vi "Autonomous Execution.vi"(8 "error in":errorcluster, 9 "Autonomous Queue":refnum<queue>, 11 "Queue Key":refnum<queue>) -> ()   [LabVIEW 2017]
uses:
  Robot Subsystems.ctl
  Drive/Drive Notifier.ctl
  Drive/Drive Control Type.ctl
  Intake/Intake Notifier.ctl
  Intake/Intake Control Type.ctl
  Intake Rotation/Intake Rotation Notifier.ctl
  Intake Rotation/Intake Rotation Control Type.ctl
  Intake Rotation/Arm Enum States.ctl
  Lift/Lift Notifier.ctl
  Lift/Lift Control Type.ctl
  Lift/Lift Enum States.ctl
  RPED/RPED Notifier.ctl
  RPED/RPED Control Type.ctl
  Queue Key Data.ctl
panel:
  in  "ignore previous (F)":bool
  in  "timeout in ms (-1)":i32=15
  out "notifiers out":refnum<notifier>[](array[refnum])
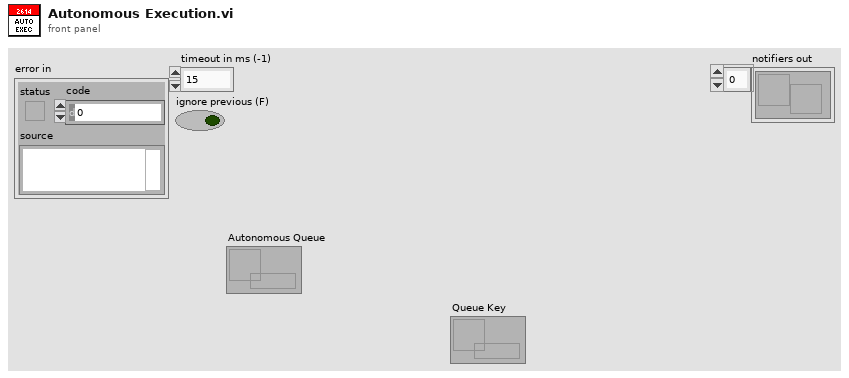
[diagram p1: front panel]
types:
  T1 = typedef "Queue Key Data.ctl" = cluster{"Operation Notifier":refnum<notifier>, "Subsystem":string, "Concurrent":bool}
  T2 = typedef "Robot Subsystems.ctl" = cluster{"Drive Notifier":T3, "Intake Notifier":T5, "Intake Rotation Notifier":T7, "Lift Notifier":T10, "RPED Notifier":T13}
  T3 = typedef "Drive Notifier.ctl" = cluster{"Drive Control Type":T4, "Throttle":dbl, "Twist":dbl, "Step":i32, "High Gear":bool, "Parameter 1":dbl, "Parameter 2":dbl, "Parameter 3":dbl, "Drive Notifier":refnum<notifier>, "AutoTrack":bool}
  T4 = typedef "Drive Control Type.ctl" = enum16{"No_Op", "Basic Drive", "Time", "Heading", "RC_Speed", "Switch_Slots", "AutoTrack_Cube", "Speed Test", "Turn_Cube", "To_Cube", "Wait", "Distance_Slow", "Distance", "Distance_Delay", "Heading_Tight", "Cube_Heading", "Distance_Ramp"}
  T5 = typedef "Intake Notifier.ctl" = cluster{"Intake Control Type":T6, "Step":i32, "In":bool, "Speed":dbl, "Out":bool, "Parameter 1":dbl, "Parameter 2":dbl, "Intake Notifier":refnum<notifier>, "Actuate Cube":bool, "Speed In":dbl, "Speed Out":dbl, "Load":bool, "Override":bool}
  T6 = typedef "Intake Control Type.ctl" = enum16{"No Op", "In", "Out", "Test Mode", "Cube_In", "Cube_Out"}
  T7 = typedef "Intake Rotation Notifier.ctl" = cluster{"Step":i32, "Intake Rotation Control Type":T8, "Parameter 1":dbl, "Parameter 2":dbl, "Intake Rotation Notifier":refnum<notifier>, "Manual Up":bool, "Manual Down":bool, "Climb":bool, "Switch":bool, "Scale Low":bool, "Scale High":bool, "Stow":bool, "Load":bool, "Scale Mid":bool, "Exchange":bool, "Set Position":T9}
  T8 = typedef "Intake Rotation Control Type.ctl" = enum16{"No Op", "Manual Up", "Position", "Manual Down", "PositionAuto"}
  T9 = typedef "Arm Enum States.ctl" = enum16{"Current Position", "Climb", "Load", "Switch", "Scale High", "Scale Mid", "Scale Low", "Exchange", "Stow"}
  T10 = typedef "Lift Notifier.ctl" = cluster{"Lift Control Type":T11, "Step":i32, "Set Position":T12, "Climb":bool, "Switch":bool, "Scale Low":bool, "Scale Mid":bool, "Scale High":bool, "Stow":bool, "Load":bool, "Climb Actuation":bool, "Manual Up":bool, "Manual Down":bool, "Parameter 1":dbl, "Parameter 2":dbl, "Parameter 3":dbl, "Lift Notifier":refnum<notifier>, "Exchange":bool, "Brake":bool}
  T11 = typedef "Lift Control Type.ctl" = enum16{"No Op", "Position", "Climb Actuation", "Manual Up", "Manual Down", "PositionAuto", "Position_Delay"}
  T12 = typedef "Lift Enum States.ctl" = enum16{"Climb", "Load", "Switch", "Scale High", "Scale Mid", "Scale Low", "Exchange", "Stow", "Current Position"}
  T13 = typedef "RPED Notifier.ctl" = cluster{"RPED Control Type":T14, "Step":i32, "Left Forward":bool, "Right Forward":bool, "Parameter 1":dbl, "Parameter 2":dbl, "Parameter 3":dbl, "RPED Notifier":refnum<notifier>, "Left Back":bool, "Right Back":bool, "Right":bool, "Left":bool}
  T14 = typedef "RPED Control Type.ctl" = enum16{"No Op", "Left Manual", "Right Manual", "Time", "Left", "Right", "Left_Slow", "Right_Slow", "Left_Distance", "Right_Distance"}
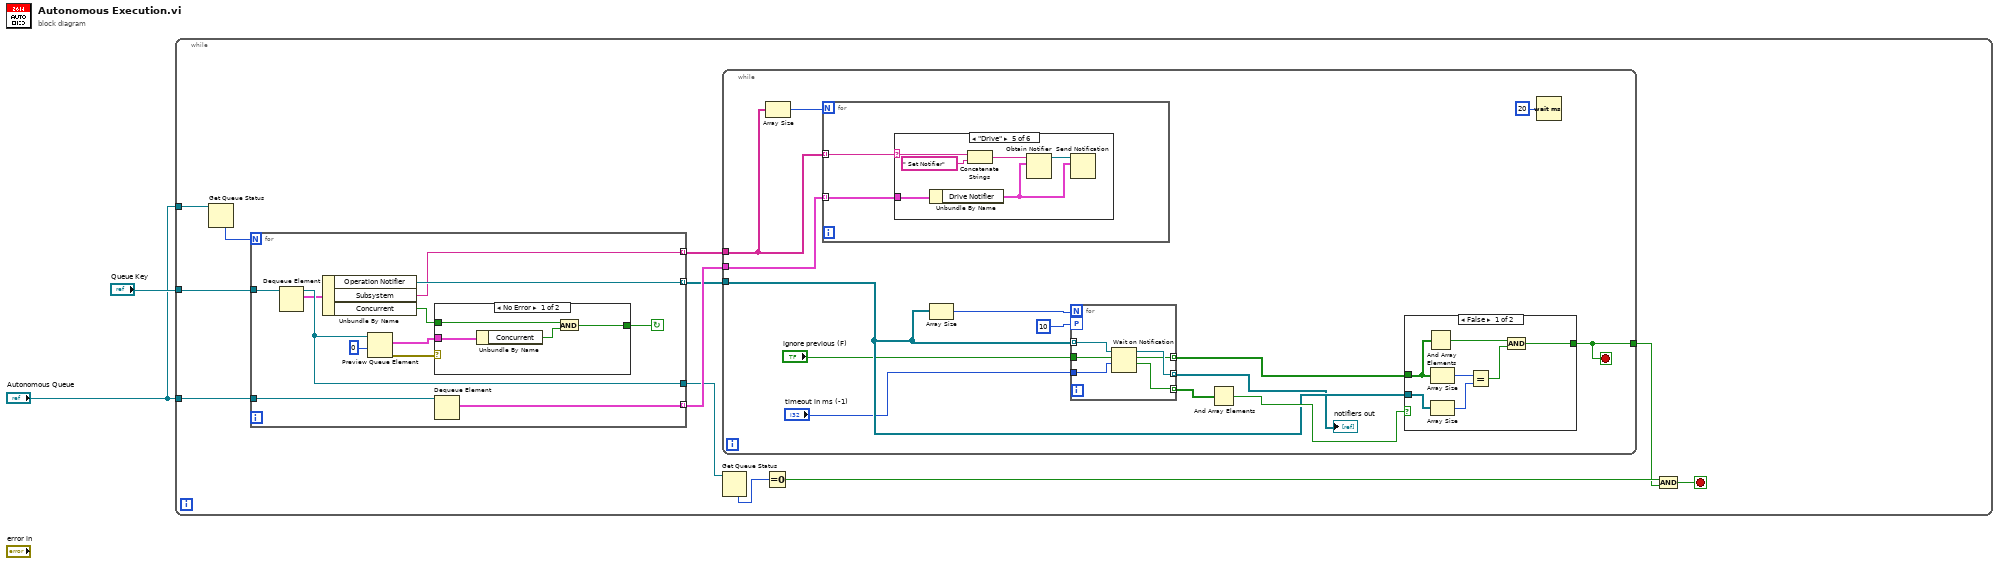
[diagram p0: block diagram]
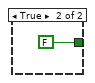
[diagram p2: hidden frame]
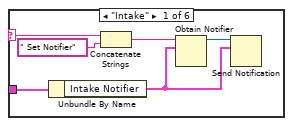
[diagram p3: hidden frame]
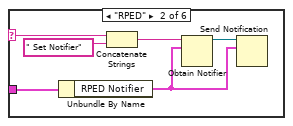
[diagram p4: hidden frame]
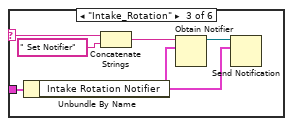
[diagram p5: hidden frame]
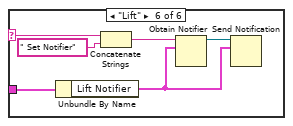
[diagram p7: hidden frame]
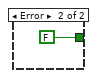
[diagram p8: hidden frame]
diagram:
  n1 = while {
    tunnel: "Queue Key" -> [w13]
    tunnel: "Autonomous Queue" -> [w14]
    tunnel: "Autonomous Queue" -> [w4]
    stop <- w6 stop-if-true
    n2 = Get Queue Status(queue=w4) -> (# elements in queue=w8:i32)  [unwired: 2 in, 7 out]
    n3 = for {
      N: w8 -> [_]
      tunnel: w14 -> [w80]
      tunnel: w13 -> [w86]
      tunnel: [w77] -> w9 mode=indexing
      tunnel: [w81] -> w3
      tunnel: [w76] -> w11 mode=indexing
      tunnel: [w79] -> w10 mode=indexing
      stop <- w82 continue-if-true
      n4 = Dequeue Element(queue=w86) -> (queue out=w81:refnum<queue>, element=w78:T1)  [unwired: 2 in, 2 out]
      n5 = Unbundle By Name(w78) -> ("Operation Notifier"=w77:refnum<notifier>, "Subsystem"=w76:string, "Concurrent"=w75:bool)
      n6 = Preview Queue Element(queue=w81, timeout in ms (-1)=0) -> (element=w85:T1, error out=w83:errorcluster)  [unwired: 1 in, 2 out]
      n7 = case shown="No Error" w83 {
        tunnel: w85 -> [w88 _]
        tunnel: [w90 FALSE] -> w82
        tunnel: w75 -> [w89 _]
        frame No Error {
          n8 = Unbundle By Name(w88) -> ("Concurrent"=w87:bool)
          n9 = And(x=w89, y=w87) -> (x .and. y?=w90:bool)
        }
        frame Error {
        }
      }
      n10 = Dequeue Element(queue=w80) -> (element=w79:T2)  [unwired: 2 in, 3 out]
    }
    n11 = while {
      tunnel: w11 -> [w23]
      tunnel: w10 -> [w22]
      tunnel: w9 -> [w24]
      tunnel: [w25] -> w5
      stop <- w25 stop-if-true
      n12 = Array Size(array=w23) -> (size(s)=w26:i32)
      n13 = for {
        N: w26 -> [_]
        tunnel: w23 -> [w44] mode=indexing
        tunnel: w22 -> [w43] mode=indexing
        n14 = case shown="\"Drive\"" w44 {
          selector: w44 -> [w48 w52 w60 _ w65 w74]
          tunnel: w43 -> [w47 w51 w59 _ w68 w73]
          frame "Intake" {
            n15 = Unbundle By Name(w47) -> ("Intake Notifier"=w49:T5)
            n16 = Concatenate Strings(w48, " Set Notifier" ("string")) -> (w46:string)
            n17 = Obtain Notifier(name (unnamed)=w46, notification data type=w49) -> (notifier out=w50:refnum<notifier>)  [unwired: 2 in, 2 out]
            n18 = Send Notification(notification=w49, notifier=w50) -> ()  [unwired: 1 in, 2 out]
          }
          frame "RPED" {
            n19 = Unbundle By Name(w51) -> ("RPED Notifier"=w55:T13)
            n20 = Concatenate Strings(w52, " Set Notifier" ("string")) -> (w56:string)
            n21 = Obtain Notifier(name (unnamed)=w56, notification data type=w55) -> (notifier out=w54:refnum<notifier>)  [unwired: 2 in, 2 out]
            n22 = Send Notification(notification=w55, notifier=w54) -> ()  [unwired: 1 in, 2 out]
          }
          frame "Intake_Rotation" {
            n23 = Unbundle By Name(w59) -> ("Intake Rotation Notifier"=w61:T7)
            n24 = Concatenate Strings(w60, " Set Notifier" ("string")) -> (w58:string)
            n25 = Obtain Notifier(name (unnamed)=w58, notification data type=w61) -> (notifier out=w62:refnum<notifier>)  [unwired: 2 in, 2 out]
            n26 = Send Notification(notification=w61, notifier=w62) -> ()  [unwired: 1 in, 2 out]
          }
          frame "No Op", Default {
          }
          frame "Drive" {
            n27 = Unbundle By Name(w68) -> ("Drive Notifier"=w66:T3)
            n28 = Concatenate Strings(w65, " Set Notifier" ("string")) -> (w64:string)
            n29 = Obtain Notifier(name (unnamed)=w64, notification data type=w66) -> (notifier out=w67:refnum<notifier>)  [unwired: 2 in, 2 out]
            n30 = Send Notification(notification=w66, notifier=w67) -> ()  [unwired: 1 in, 2 out]
          }
          frame "Lift" {
            n31 = Unbundle By Name(w73) -> ("Lift Notifier"=w71:T10)
            n32 = Concatenate Strings(w74, " Set Notifier" ("string")) -> (w70:string)
            n33 = Obtain Notifier(name (unnamed)=w70, notification data type=w71) -> (notifier out=w72:refnum<notifier>)  [unwired: 2 in, 2 out]
            n34 = Send Notification(notification=w71, notifier=w72) -> ()  [unwired: 1 in, 2 out]
          }
        }
      }
      n35 = Array Size(array=w24) -> (size(s)=w18:i32)
      n36 = for {
        N: w18 -> [_]
        tunnel: w24 -> [w34] mode=indexing
        workers-P: 10 -> [_]
        tunnel: "timeout in ms (-1)" -> [w33]
        tunnel: "ignore previous (F)" -> [w32]
        tunnel: [w31] -> w21 mode=indexing
        tunnel: [w30] -> w28 mode=indexing
        tunnel: [w29] -> w16 mode=indexing
        n37 = Wait on Notification(notifier=w34, ignore previous (F)=w32, timeout in ms (-1)=w33) -> (notifier out=w31:refnum<notifier>, notification=w30:bool, timed out?=w29:bool)  [unwired: 1 in, 1 out]
      }
      "notifiers out" <- w21
      n38 = And Array Elements(Boolean array=w16) -> (logical AND=w27:bool)
      n39 = case shown="False" w27 {
        tunnel: [w40 FALSE] -> w25
        tunnel: w28 -> [w39 _]
        tunnel: w24 -> [w38 _]
        frame False {
          n40 = And Array Elements(Boolean array=w39) -> (logical AND=w41:bool)
          n41 = Array Size(array=w39) -> (size(s)=w37:i32)
          n42 = Array Size(array=w38) -> (size(s)=w36:i32)
          n43 = Equal?(x=w37, y=w36) -> (x = y?=w35:bool)
          n44 = And(x=w41, y=w35) -> (x .and. y?=w40:bool)
        }
        frame True {
        }
      }
      n45 = Wait (ms)(milliseconds to wait=u32 20) -> ()  [unwired: 1 out]
    }
    n46 = Get Queue Status(queue=w3) -> (# elements in queue=w12:i32)  [unwired: 2 in, 7 out]
    n47 = Equal To 0?(x=w12) -> (x = 0?=w7:bool)
    n48 = And(x=w7, y=w5) -> (x .and. y?=w6:bool)
  }
